vi "About.vi"() -> ()   [LabVIEW 2020, in "XMenuBar.xctl"]
doc: "Use this template to create a dialog box with event handling."
uses:
  XMenuBar.xctl
panel:
  in  "OK":bool
  # "XMenu Bar\nVERSION: 1.0\n2010-Sept.\nBy Hightech"
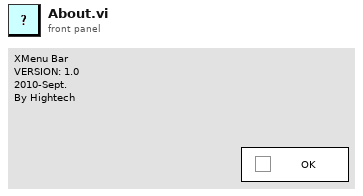
[diagram p1: front panel]
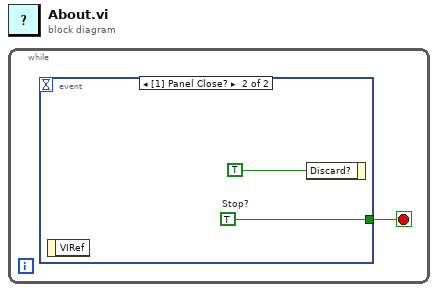
[diagram p0: block diagram]
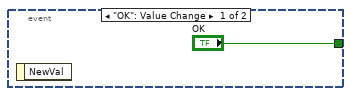
[diagram p2: hidden frame]
diagram:
  n1 = while {
    stop <- w1 stop-if-true
    n2 = event shown="[1] Panel Close?" {
      selector: _ -> [_ _]
      dyn-events: _ -> [_ _]
      timeout: _ -> [_ _]
      tunnel: ["OK" w3] -> w1
      event "OK": Value Change {
        n3 = event-data() -> ()  [unwired: 1 in, 1 out]
      }
      event Panel Close? {
        w3 = TRUE  # Stop?
        n4 = event-data() -> ()  [unwired: 1 in, 1 out]
        n5 = event-data("Discard?"=TRUE) -> ()  [unwired: 1 in, 1 out]
      }
    }
  }
